vi "Teardown.vi"(8 "error in (no error)":errorcluster, 11 "Bus Controller in":refnum<class "Bus Controller.lvclass">) -> (0 "error out":errorcluster)   [LabVIEW 2020, in "Unit Tests.lvlib" / "Bus Controller.lvclass"]
uses:
  Bus Controller.lvclass
  Utilities/Simulated FPGA/FPGA Sim.lvclass
  Bus Controller.lvclass/Bus Controller.ctl
  <vilib>/Utility/error.llb/Clear Errors.vi
  1553 Session/1553 Session.lvclass
  Dependencies/Registry/Registry.lvclass
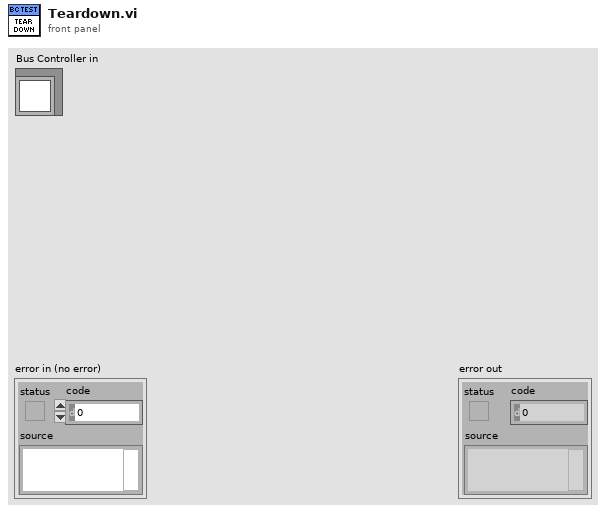
[diagram p1: front panel]
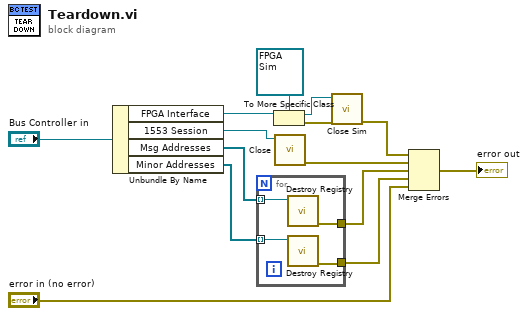
[diagram p0: block diagram]
diagram:
  n1 = Unbundle By Name("Bus Controller in") -> ("FPGA Interface"=w14:refnum<class "FPGA Interface.lvclass">, "1553 Session"=w7:refnum<class "1553 Session.lvclass">, "Msg Addresses"=w5:refnum<class "Registry.lvclass">[], "Minor Addresses"=w4:refnum<class "Registry.lvclass">[])
  n2 = for {
    tunnel: w5 -> [w18] mode=indexing
    tunnel: w4 -> [w17] mode=indexing
    tunnel: [w16] -> w3
    tunnel: [w15] -> w2
    n3 = call "Destroy Registry.vi"("Registry in"=w18) -> ("error out"=w16:errorcluster)  [unwired: 7 in, 3 out]
    n4 = call "Destroy Registry.vi"("Registry in"=w17) -> ("error out"=w15:errorcluster)  [unwired: 7 in, 3 out]
  }
  n5 = To More Specific Class(target class=refnum<class "FPGA Sim.lvclass"> refnum ("FPGA Sim.lvclass"), reference=w14) -> (specific class reference=w12:refnum<class "FPGA Sim.lvclass">, error out=w11:errorcluster)  [unwired: 1 in]
  n6 = call-dynamic "Close.vi"("1553 Board in"=w7) -> ("error out"=w6:errorcluster)  [unwired: 10 in]
  n7 = call "Close Sim.vi"("error in (no error)"=w11, "FPGA Sim in"=w12) -> ("error out"=w10:errorcluster)  [unwired: 9 in]
  n8 = Merge Errors(w10, w6, w3, w2, "error in (no error)") -> (→"error out":errorcluster)
